vi "Greteer.vi"(8 "error in":errorcluster) -> (0 "error out":errorcluster, 3 "Exercise Folder Path":path)   [LabVIEW 2014]
uses:
  <vilib>/Utility/miscctls.llb/LVPointTypeDef.ctl
panel:
  in  "close":bool
  # "Tutorial 3 - Exercício de LabVIEW"
  # "Este programa é um exercício da disciplina PSI3214 - Laboratório de Instrumentação Eletrica, e visa fixar os conceitos vistos no tutorial 3. Neste execício queremos projetar um sistema de aquisição de dados, levando em conta não só as características temporais de um sinal, visto no tutorial 2, como também sua caracterização no domínio da frequência. O programa deste exercício foi montado para que tenha as mesmas funcionalidades vistas e programadas durante os exemplos do tutorial. Sendo assim, faça uso do documento em pdf fornecido para realização deste exercício, caso julgue necessário. \n\n{Como funciona o exercício}\n - Você terá os Exercícios 3.1 e 3.2 a serem realizados \n - Para começar um exercício voce deve clicar no icone gerar sinal, correspondente ao exercício desejado\n\n\n\n\n\n\n\n\n - Feita a etapa acima, você verá no gráfico principal o sinal correspondente ao exercício selecionado\n\n\n\n\n\n\n\n\n\n\n\n\n\n\n\n\n\n\n\n - Após isso você deverá clicar no Enunciado do exercicio correspondente e uma tela será aberta com o enunciado de cada exercicio\n\n\n\n\n\n\n\n\n\n - Todos os exercícios desta série de tutoriais possuem campos os quais deverão ser preenchidos. Em campos cuja resposta esperada é um número, a resposta do aluno deverá se encontrar em uma margem de +-5% do valor verdadeiro para que seja considerada correta. \n\n\n\n\n\n\n\n\n\n\n- Note que como o intuito do exercício é de que seja priorizado o aprendizado do aluno, você terá quantas tentativas desejar para completar o exercício. Use os controles disponíveis no painel principal do VI ex3.vi para atuar sobre o sinal gerado e faça uso das diferentes visualizações do sinal (domínio do tempo e da frequêcia) por meio do menu \"Change Graph View\" para analizar o sinal.\n\n\n\n\n\n\n\n\n\n\n\n\n\n\n\n\n\n- Para fechar o enunciado e voltar à tela principal acione o botão \"Close Form\". Note que todas as respostas serão salvas e serão mostradas na proxima vez que abrir o enunciado!\n\n\n\n\n\n\n\n\n\n\n\n - Após 70% das tarefas do enunciado sejam completadas, o ícone de interrogação será habilitado. Nele você poderá verificar quais respostas estão corretas. \n\n\n\n\n\n\n\n\n\n\n\n - Depois de acabados os exercicios clique no botão stop para sair do programa\n - Você deverá responder um formulário de avaliação dos tutoriais\n - Ao final do exercício você terá alguns arquivos na pasta \".../Tutorial 1/Exercises/moodle_files/\". Como última tarefa você deverá submeter essas tarefas no Moodle USP.\n\n\n\n\n\n\n\n\n\n\n\n\n\n\n\n\n- Em caso de algum erro inesperado, tente reiniciar o LabVIEW. Caso ainda ocorram problemas contate o professor responsável pelo curso!\n\nTanto os resultados, quanto o desempenho neste exercício serão utilizados para melhorar a disciplina em anos futuros, deste modo, no formulário de término do exercício faça comentários que ache pertinente em relação aos tutoriais da disciplina. Bom exercício!"
  # "Fig. i.1 - Botão \"Gerar Sinal\""
  # "Fig. i.2 - Botão \"Gerar Sinal\" Acionado"
  # "Fig. i.3 - Sinal no painel principal"
  # "Fig. i.4 - Botão \"Enunciado\", em destaque"
  # "Fig. i.5 - Tolerância da Resposta"
  # "Fig. i.6 - Controles do Painal Frontal do Exercício"
  # "Fig. i.7 - Controles de visualização do sinal"
  # "Fig. i.8 - Campos de preenchimento dentro de um exercício"
  # "Fig. i.9 - Botão \"Close Form\""
  # "Fig. i.10 - Indicador de percentual do exercício que foi respondido"
  # "Fig. i.12 - Campos após correção automática"
  # "Fig. i.11 - Botão \"?\""
  # "report.txt"
  # "tut3ex1.png"
  # "tut3eval.png"
  # "tut3ex2.png"
  # "Fig. i.13 - Upload de Arquivos no Moodle"
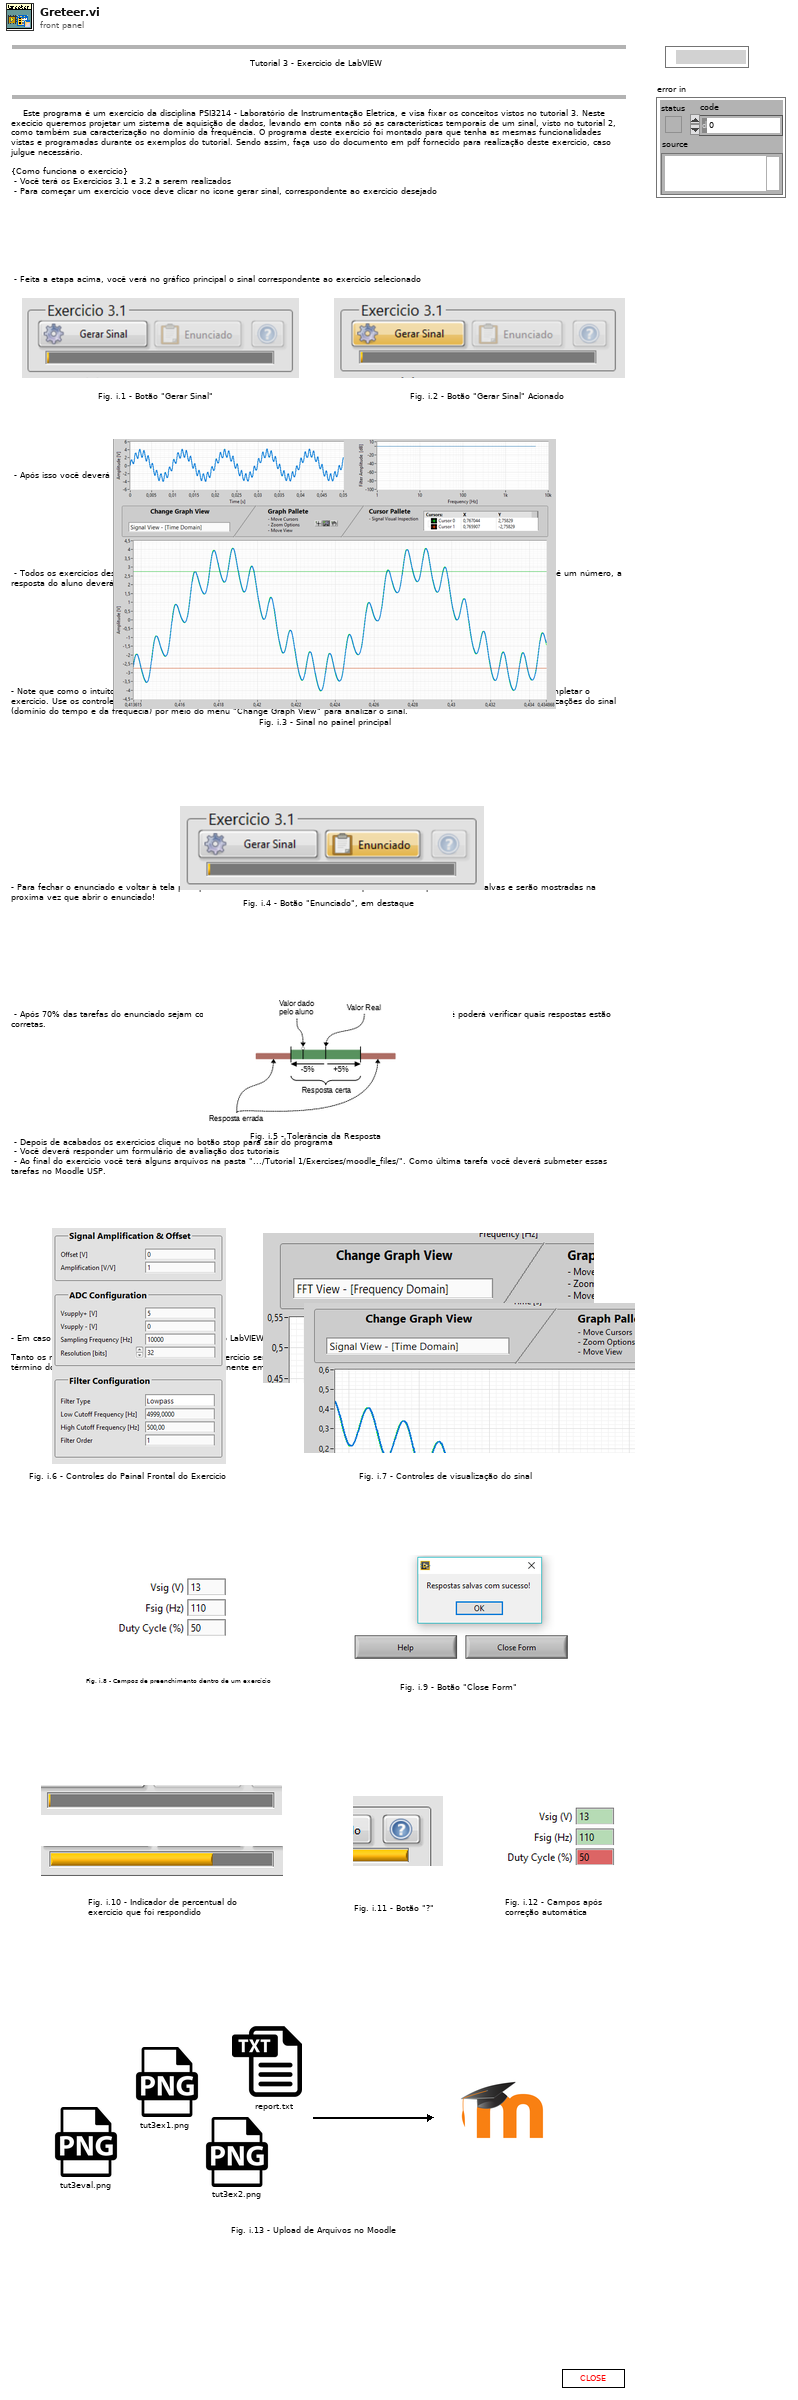
[diagram p1: front panel]
types:
  T1 = typedef "LVPointTypeDef.ctl" = cluster{"Horizontal":i16, "Vertical":i16}
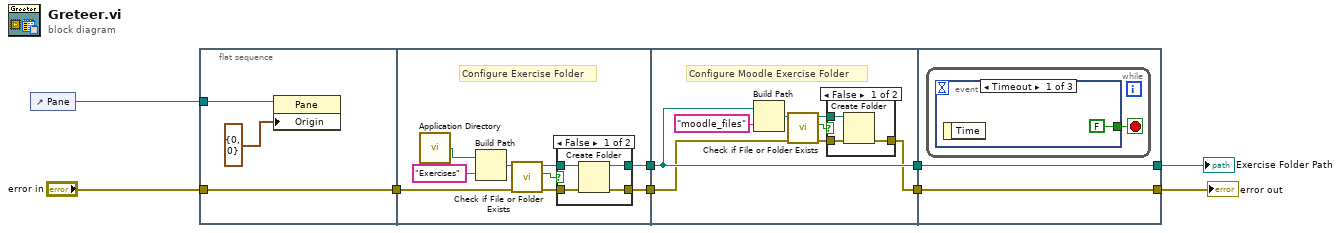
[diagram p0: block diagram]
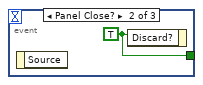
[diagram p4: hidden frame]
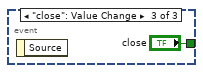
[diagram p5: hidden frame]
diagram:
  n1 = control-ref of="Pane"() -> (w6:refnum<vi>)
  n2 = flat-sequence {
    tunnel: "error in" -> [w12]
    tunnel: [w12] -> w7
    tunnel: w6 -> [w11]
    tunnel: [w16] -> w4
    tunnel: [w15] -> w2
    tunnel: w7 -> [w14]
    tunnel: w4 -> [w30]
    tunnel: [w30] -> w3
    tunnel: w2 -> [w29]
    tunnel: [w28] -> w1
    tunnel: [w40] -> w5
    tunnel: [w41] -> w9
    tunnel: w3 -> [w41]
    tunnel: w1 -> [w40]
    frame #0 {
      n3 = property class="Pane"(reference=w11, "Origin"=T1 {"Horizontal"=0, "Vertical"=0}) -> ()  [unwired: 1 in, 2 out]
    }
    frame #1 {
      # "Configure Exercise Folder"
      n4 = call <vilib>:"Application Directory.vi"() -> ("Application Directory"=w21:path)
      n5 = Build Path(base path=w21, name or relative path="Exercises") -> (appended path=w18:path)
      n6 = call <vilib>:"Check if File or Folder Exists.vi"("error in (no error)"=w14, "path"=w18) -> ("error out"=w17:errorcluster, "file or folder exists?"=w19:bool, "dup path"=w13:path)  [unwired: 7 in]
      n7 = case shown="False" w19 {
        tunnel: w13 -> [w25 w27]
        tunnel: w17 -> [w24 w26]
        tunnel: [w23 w27] -> w16
        tunnel: [w22 w26] -> w15
        frame False {
          n8 = Create Folder(path (use dialog)=w25, error in=w24) -> (created path=w23:path, error out=w22:errorcluster)  [unwired: 1 in, 1 out]
        }
        frame True {
        }
      }
    }
    frame #2 {
      # "Configure Moodle Exercise Folder"
      n9 = Build Path(base path=w30, name or relative path="moodle_files") -> (appended path=w33:path)
      n10 = call <vilib>:"Check if File or Folder Exists.vi"("error in (no error)"=w29, "path"=w33) -> ("error out"=w32:errorcluster, "file or folder exists?"=w34:bool, "dup path"=w31:path)  [unwired: 7 in]
      n11 = case shown="False" w34 {
        tunnel: w31 -> [w38 _]
        tunnel: w32 -> [w37 w39]
        tunnel: [w36 w39] -> w28
        frame False {
          n12 = Create Folder(path (use dialog)=w38, error in=w37) -> (error out=w36:errorcluster)  [unwired: 1 in, 2 out]
        }
        frame True {
        }
      }
    }
    frame #3 {
      n13 = while {
        stop <- w42 stop-if-true
        n14 = event shown="[0] Timeout" {
          selector: _ -> [_ _ _]
          dyn-events: _ -> [_ _ _]
          timeout: _ -> [_ _ _]
          tunnel: [FALSE ("close") w44 "close"] -> w42
          event Timeout {
            n15 = event-data() -> ()  [unwired: 1 in, 1 out]
          }
          event Panel Close? {
            w44 = TRUE ("Discard?")
            n16 = event-data() -> ()  [unwired: 1 in, 1 out]
            n17 = event-data("Discard?"=w44) -> ()  [unwired: 1 in, 1 out]
          }
          event "close": Value Change {
            n18 = event-data() -> ()  [unwired: 1 in, 1 out]
          }
        }
      }
    }
  }
  "Exercise Folder Path" <- w9
  "error out" <- w5
